vi "Update Detector Voltage.vi"(4 "HasESI2":bool=TRUE, 5 "HasESI1":bool=TRUE) -> (0 "Proceed":bool, 1 "Run Auto-Detector Bias Procedure":bool)   [LabVIEW 2015]
uses:
  Type/_RT Command.ctl
  <vilib>/Utility/config.llb/Read Key (Path).vi
  <vilib>/Utility/config.llb/NI_LVConfig.lvlib
panel:
  in  "Optimize":bool
  out "FileNames":path[](array[path])
  in  "Quit":bool
  in  "UserInput":dbl=2000.0
  in  "Select":bool
  in  "Cancel":bool
  # "Please enter the desired detector voltage\nor click Optimize to run the Auto-Detector optimization algorithm"
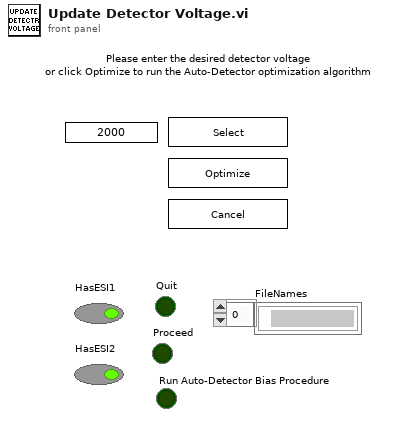
[diagram p1: front panel]
types:
  T1 = typedef "NI_LVConfig.lvlib/Config Data RefNum.ctl" = refnum<k1>
  T2 = typedef "_GUI Method.ctl" = cluster{"Lenses":T3[], "Mass Ranges":T4[], "Acquire":bool, "MCA":bool, "Q1DC EN":bool, "Q1 POL":bool, "Q3 POL":bool, "Q1 RF  EN":bool, "Averaging":bool, "Log Scale":bool, "CPS":bool, "Unit":bool, "Data Path":path, "Run Mode":T7, "Fixed Mass (amu)":dbl, "Q3DC EN":bool, "Q3 RF  EN":bool, "Negative":bool}
  T3 = typedef "_Lens Property.ctl" = cluster{"Scan Type":u8, "Scans":i32, "Time 1":dbl, "Time 2":dbl, "Value 1":dbl, "Value 2":dbl, "Step Size":dbl}
  T4 = typedef "_Mass Range Property.ctl" = cluster{"Start":dbl, "Stop":dbl, "Step Size":dbl, "Steps":i32, "Dwell":dbl, "Parameters":T5[], "Res":T6}
  T5 = typedef "_Mass Range Parameters.ctl" = cluster{"Name":string, "Ch#":u8, "StartV":dbl, "StopV":dbl, "StepV":dbl, "Index":u8}
  T6 = typedef "_RT Res Type.ctl" = u16
  T7 = typedef "_Run Mode.ctl" = enum16{"MRM (Q1/Q2)", "Q1 Scan", "Q1 SRM", "Q2 Scan", "Q2 SRM", "Product Scan", "Precursor Scan", "Neutral Loss", "Neutral Gain"}
  T8 = typedef "_RT Command.ctl" = enum16{"xml Start Run", "xml Start Actual Run", "xml Stop Run", "xml Runtime Update", "xml Get Status", "xml Get Table", "xml Set Table", "xml Get Configuration", "xml System Status", "xml Set LC Input Logic", "xml Get Data", "xml Get Info", "Start", "StartActualRun", "Stop", "Runtime Update", "Get Data", "Get Info", "Get Status", "Get Param", "Get Config", "Get Table", "Read ADC", "Set Oscillator", "Update Config", "Update Table", "Set All Pol", "Set Pol and DC", "Set Max Mass", "Toggle RP", "Toggle EL", "Set PIC", "Initialize Turbo", "Send Turbo Comm", "Close Turbo", "P1", "P2", "P3", "Send Serial", "Set LC Out", "Get LC In", "Read VAC", "Test Table", "Toggle Power", "Get Startup", "Set Startup", "Get ADC Table", "Set ADC Table", "Get Brief Status", "Get Detail Status", "Auxiliary Update", "Set CC Logics", "Set CC Input Logics", "Ignore Error", "invalid"}
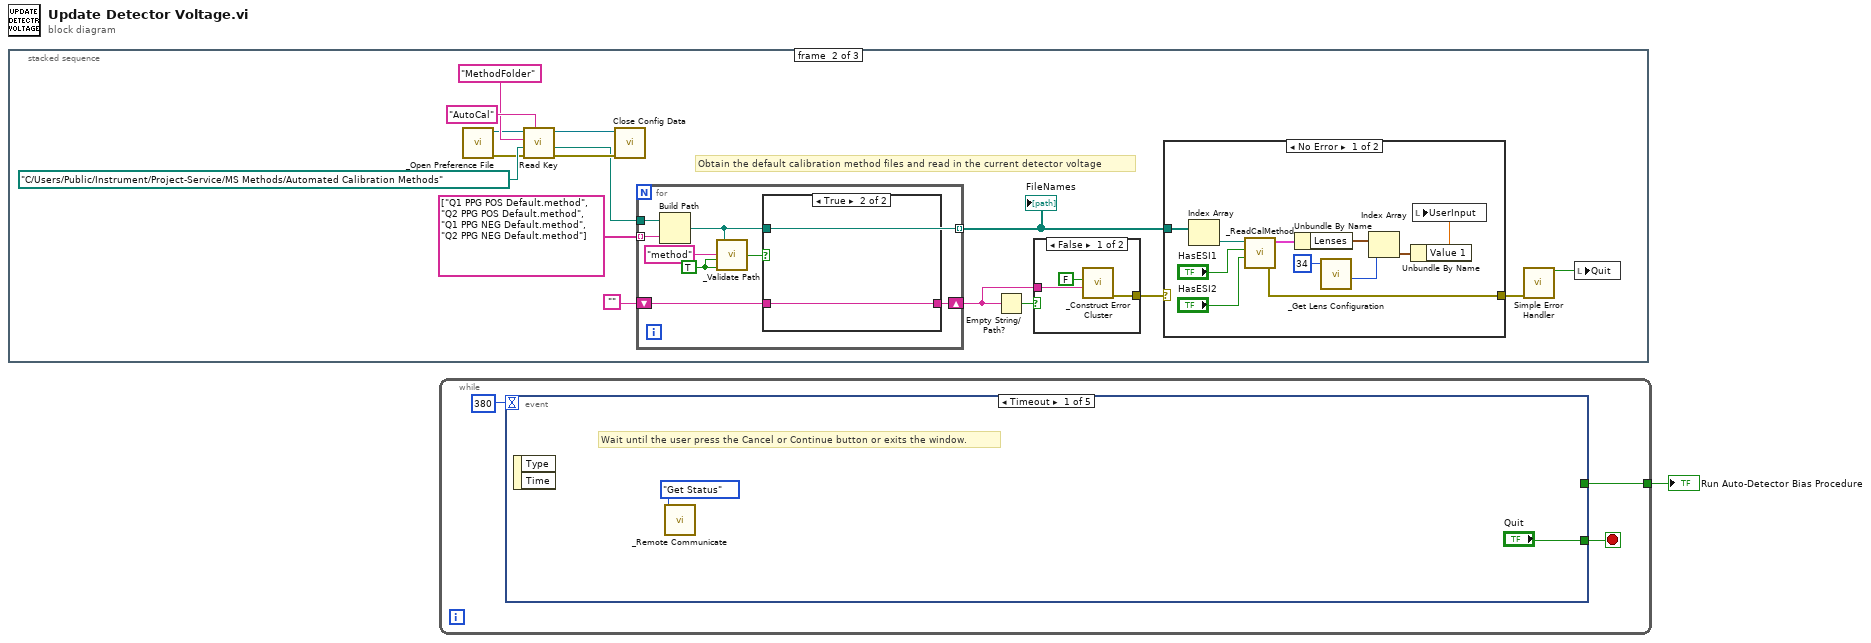
[diagram p0: block diagram]
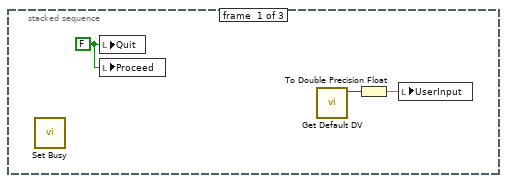
[diagram p2: hidden frame]
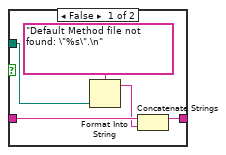
[diagram p5: hidden frame]
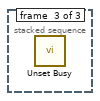
[diagram p6: hidden frame]
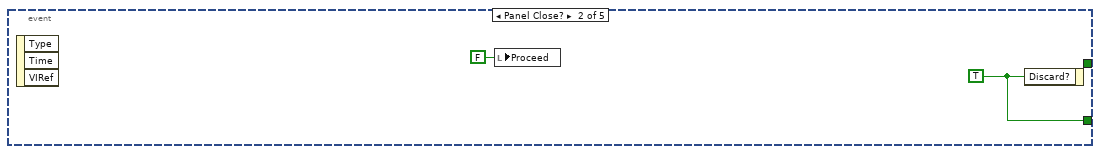
[diagram p7: hidden frame]
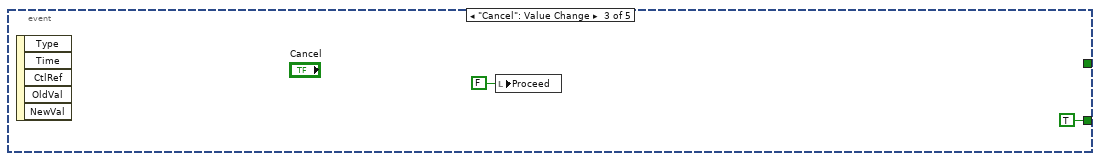
[diagram p8: hidden frame]
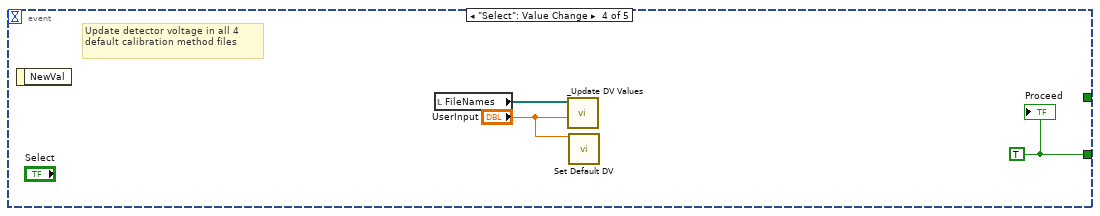
[diagram p9: hidden frame]
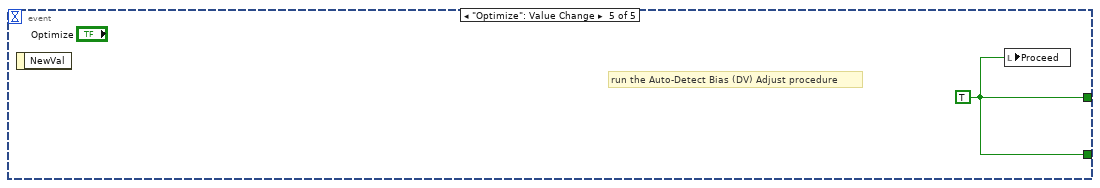
[diagram p10: hidden frame]
diagram:
  n1 = stacked-sequence {
    frame #0 {
      w4 = FALSE ("Quit")
      n2 = call <vilib>:"Set Busy.vi"() -> ()  [unwired: 10 in, 2 out]
      n3 = local write "Quit"(w4) -> ()
      n4 = local write "Proceed"(w4) -> ()
      n5 = call "Get Default DV.vi"() -> ("DV Default Value"=w3:i32)  [unwired: 10 in, 1 out]
      n6 = To Double Precision Float(number=w3) -> (double precision float=w2:dbl)
      n7 = local write "UserInput"(w2) -> ()
    }
    frame #1 {
      # "Obtain the default calibration method files and read in the current detector voltage"
      n8 = call "_Open Preference File.vi"() -> ("error"=w10:errorcluster, "refnum"=w8:T1)  [unwired: 3 in, 3 out]
      n9 = call-poly <vilib>:"Read Key.vi"("section"="AutoCal", "error in (no error)"=w10, "default value"=path "C:/Users/Public/Instrument/Project-Service/MS Methods/Automated Calibration Methods" ("oldTablePath"), "key"="MethodFolder" ("section"), "refnum"=w8) -> ("error out"=w6:errorcluster, "value"=w5:path, "refnum out"=w7:T1)  [unwired: 3 in, 1 out]
      n10 = call <vilib>:"Close Config Data.vi"("error in (no error)"=w6, "refnum"=w7) -> ()  [unwired: 8 in, 2 out]
      n11 = for {
        tunnel: string[] ["Q1 PPG POS Default.method", "Q2 PPG POS Default.method", "Q1 PPG NEG Default.method", "Q2 PPG NEG Default.method"] -> [w43] mode=indexing
        tunnel: w5 -> [w42]
        tunnel: [w38] -> w15 mode=indexing
        shift-right: [w36] -> w17
        shift-left: "" -> [w37]
        w40 = TRUE ("Check Type (F)")
        n12 = Build Path(base path=w42, name or relative path=w43) -> (appended path=w38:path)
        n13 = call "_Validate Path.vi"("Check Type (F)"=w40, "Check Exist (F)"=w40, "Type (isd)"="method", "path"=w38) -> ("Valid"=w39:bool)
        n14 = case shown="True" w39 {
          tunnel: w38 -> [w48 _]
          tunnel: w37 -> [w46 w49]
          tunnel: [w44 w49] -> w36
          frame False {
            n15 = Format Into String(format string="Default Method file not found: \"%s\".\n", w48) -> (resulting string=w45:string)  [unwired: 2 in, 1 out]
            n16 = Concatenate Strings(w46, w45) -> (w44:string)
          }
          frame True {
          }
        }
      }
      "FileNames" <- w15
      n17 = Empty String/Path?(string/path=w17) -> (empty?=w18:bool)
      n18 = case shown="False" w18 {
        tunnel: w17 -> [w34 _]
        tunnel: [w33 _] -> w16
        frame False {
          n19 = call "_Construct Error Cluster.vi"("reason"=w34, "CallingChain? (T)"=FALSE) -> ("error out"=w33:errorcluster)  [unwired: 5 in]
        }
        frame True {
        }
      }
      n20 = case shown="No Error" w16 {
        selector: w16 -> [_ w32]
        tunnel: w15 -> [w31 _]
        tunnel: [w26 w32] -> w14
        frame No Error {
          n21 = Index Array(array=w31) -> (element=w30:path)  [unwired: 1 in]
          n22 = call "_ReadCalMethod.vi"("HasESI2"="HasESI2", "HasESI1"="HasESI1", "Method Path"=w30) -> ("error out"=w26:errorcluster, "GUI Method"=w27:T2)  [unwired: 2 in, 1 out]
          n23 = Unbundle By Name(w27) -> ("Lenses"=w23:T3[])
          n24 = call "_Get Lens Configuration.vi"("Channel #"=u8 34) -> ("Config Row#"=w22:i32)  [unwired: 1 in, 5 out]
          n25 = Index Array(array=w23, index=w22) -> (element=w24:T3)
          n26 = Unbundle By Name(w24) -> ("Value 1"=w21:dbl)
          n27 = local write "UserInput"(w21) -> ()
        }
        frame Error {
        }
      }
      n28 = call <vilib>:"Simple Error Handler.vi"("error in (no error)"=w14) -> ("error?"=w13:bool)  [unwired: 4 in, 4 out]
      n29 = local write "Quit"(w13) -> ()
    }
    frame #2 {
      n30 = call <vilib>:"Unset Busy.vi"() -> ()  [unwired: 11 in, 1 out]
    }
  }
  n31 = while {
    tunnel: [w50] -> w1
    stop <- w51 stop-if-true
    n32 = event shown="[0] Timeout" {
      selector: _ -> [_ _ _ _ _]
      dyn-events: _ -> [_ _ _ _ _]
      timeout: 380 -> [_ _ _ _ _]
      tunnel: ["Quit" w56 TRUE ("Discard?") w61 w62] -> w51
      tunnel: [_ _ _ _ w62] -> w50
      event Timeout {
        # "Wait until the user press the Cancel or Continue button or exits the window."
        n33 = event-data() -> ()  [unwired: 1 in, 2 out]
        n34 = call "_Remote Communicate.vi"("Command"=_RT_Command."Get Status") -> ()  [unwired: 5 in, 4 out]
      }
      event Panel Close? {
        w56 = TRUE ("Discard?")
        n35 = event-data() -> ()  [unwired: 1 in, 3 out]
        n36 = local write "Proceed"(FALSE ("Proceed")) -> ()
        n37 = event-data("Discard?"=w56) -> ()  [unwired: 1 in, 1 out]
      }
      event "Cancel": Value Change {
        n38 = event-data() -> ()  [unwired: 1 in, 5 out]
        n39 = local write "Proceed"(FALSE ("Proceed")) -> ()
      }
      event "Select": Value Change {
        w61 = TRUE ("Discard?")
        # "Update detector voltage in all 4 default calibration method files"
        n40 = event-data() -> ()  [unwired: 1 in, 1 out]
        n41 = local read "FileNames"() -> (w60:path[])
        n42 = call "_Update DV Values.vi"("UserInput"="UserInput", "FileNames"=w60) -> ()  [unwired: 9 in, 1 out]
        n43 = call "Set Default DV.vi"("DV Default Value"="UserInput") -> ()  [unwired: 10 in, 1 out]
        "Proceed" <- w61
      }
      event "Optimize": Value Change {
        w62 = TRUE ("Optimize")
        # "run the Auto-Detect Bias (DV) Adjust procedure"
        n44 = event-data() -> ()  [unwired: 1 in, 1 out]
        n45 = local write "Proceed"(w62) -> ()
      }
    }
  }
  "Run Auto-Detector Bias Procedure" <- w1
